vi "SoundCalibration.vi"(9 "通道号":i32, 10 "通道选择":enum16{"通道1", "通道2", "通道3", "通道4"}(ring), 11 "设备选择":refnum<visa-resource-name>) -> ()   [LabVIEW 2020, in "bas_meas.lvlib"]
uses:
  bas_meas.lvlib
panel:
  in  "取消":bool
  out "已排序的数组":string[](array[string])
  out "选中通道":string
  out "校准状态":string
  out "x-y":dbl
  out "数值":dbl
  out "结果字符串":string
  out "read buffer":string
  in  "校准声级(dB)":dbl=94.0 format="%.2g"
  out "SPL(dB)":dbl format="%.2f"
  in  "校准":bool
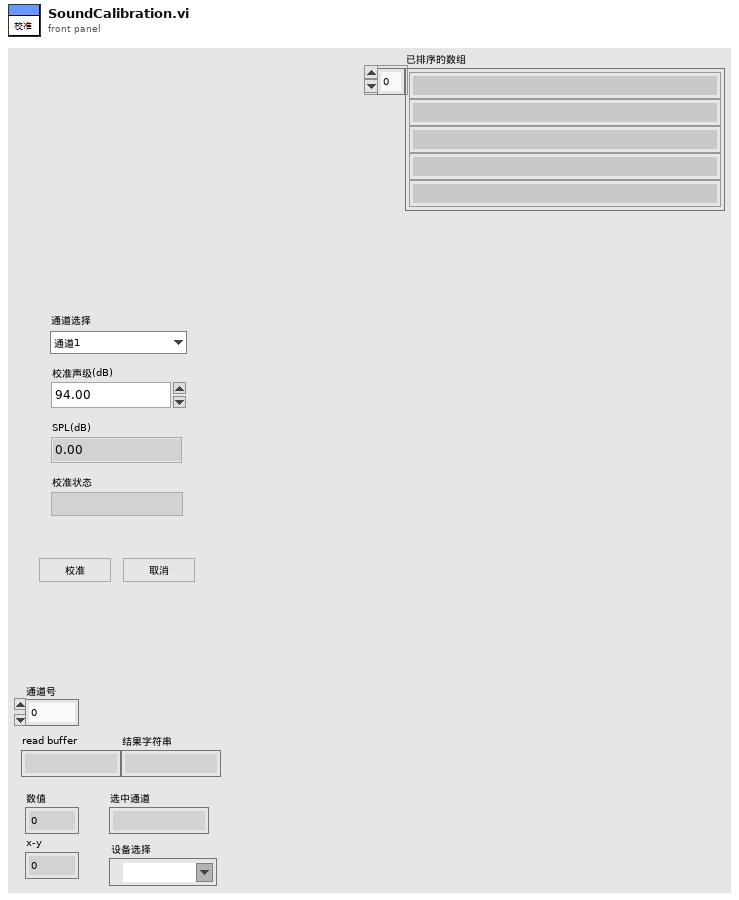
[diagram p1: front panel]
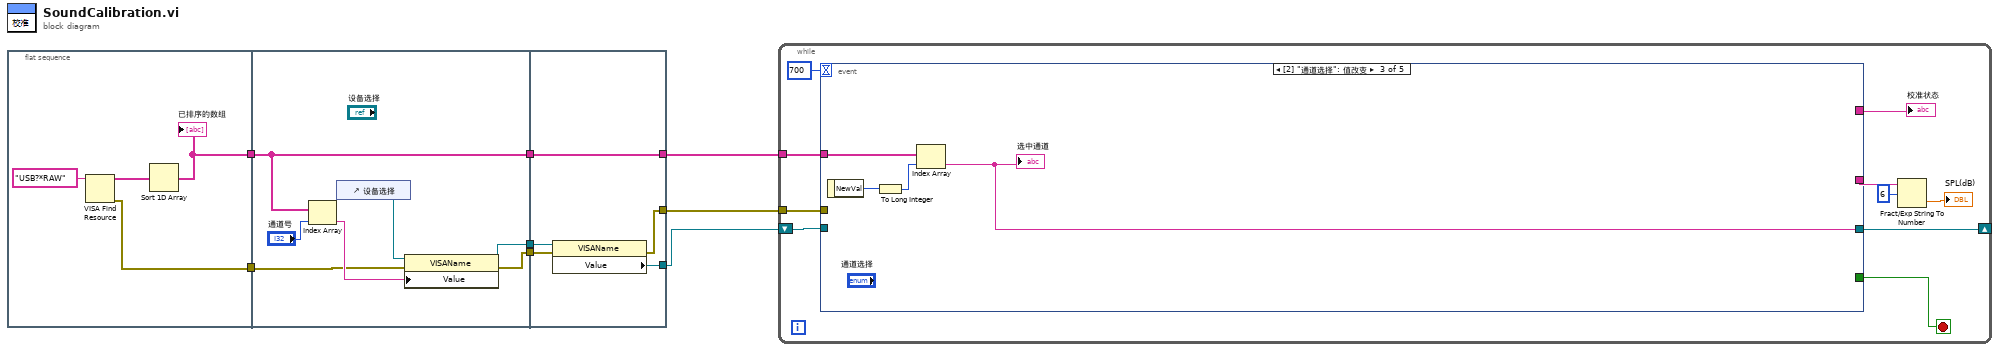
[diagram p0: block diagram]
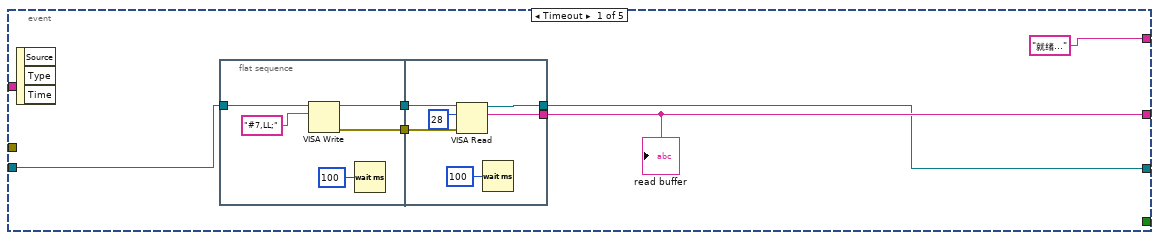
[diagram p2: hidden frame]
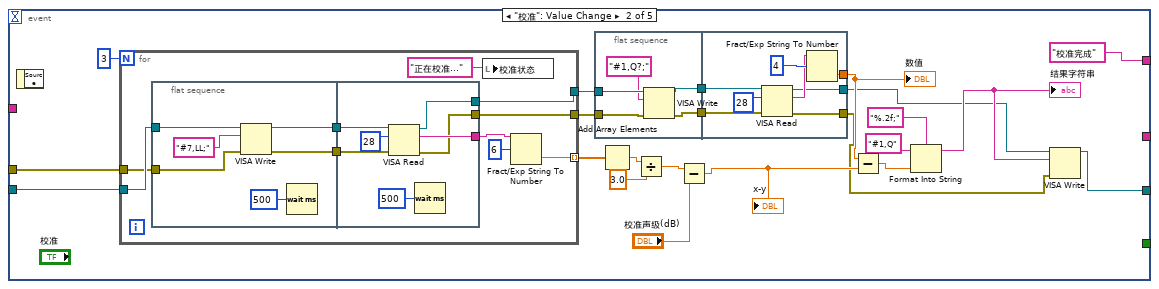
[diagram p3: hidden frame]
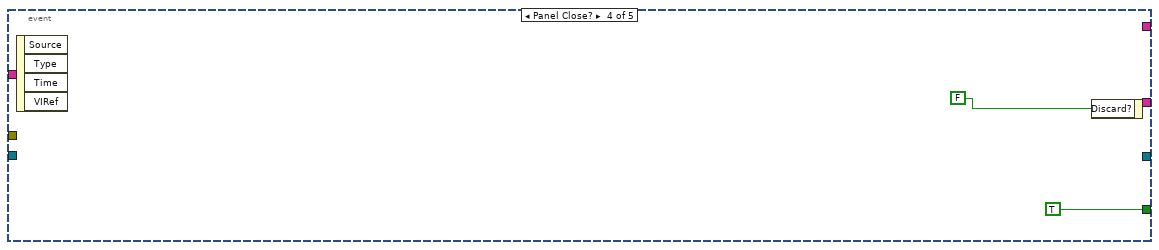
[diagram p4: hidden frame]
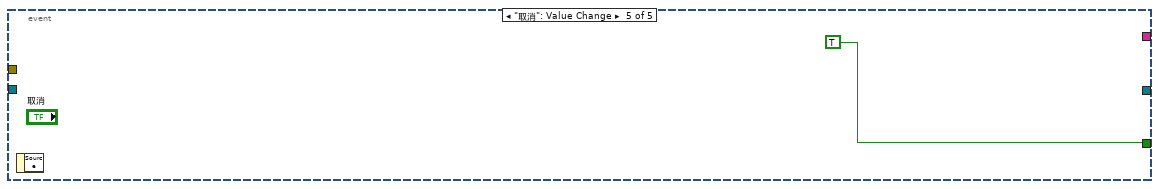
[diagram p5: hidden frame]
diagram:
  n1 = flat-sequence {
    tunnel: [w10] -> w7
    tunnel: [w9] -> w2
    tunnel: w7 -> [w19]
    tunnel: [w19] -> w6
    tunnel: [w16] -> w5
    tunnel: [w15] -> w4
    tunnel: w2 -> [w14]
    tunnel: [w24] -> w8
    tunnel: w6 -> [w24]
    tunnel: w5 -> [w23]
    tunnel: w4 -> [w22]
    tunnel: [w21] -> w3
    tunnel: [w20] -> w1
    frame #0 {
      n2 = VISA Find Resource(11:"USB?*RAW" ("表达式(\"?*\")")) -> (0:w9:errorcluster, 3:w11:string[])  [unwired: 2 in, 1 out]
      n3 = Sort 1D Array(array=w11) -> (sorted array=w10:string[])
      "已排序的数组" <- w10
    }
    frame #1 {
      n4 = Index Array(array=w19, index="通道号") -> (element=w18:string)
      n5 = control-ref of="设备选择"() -> (w17:refnum<vi>)
      n6 = property class="VISAName"(reference=w17, error in=w14, "Value"=w18) -> (reference out=w16:refnum<vi>, error out=w15:errorcluster)
    }
    frame #2 {
      n7 = property class="VISAName"(reference=w23, error in=w22) -> (error out=w20:errorcluster, "Value"=w21:refnum<visa-resource-name>)  [unwired: 1 out]
    }
  }
  n8 = while {
    tunnel: w8 -> [w27]
    shift-right: [w26] -> _
    shift-left: w3 -> [w33]
    tunnel: w1 -> [w25]
    stop <- w34 stop-if-true
    n9 = event shown="[2] \"通道选择\": 值改变" {
      selector: _ -> [_ _ _ _ _]
      dyn-events: _ -> [_ _ _ _ _]
      timeout: 700 -> [_ _ _ _ _]
      tunnel: [_ _ _ TRUE ("放弃？") TRUE ("放弃？")] -> w34
      tunnel: w33 -> [w38 w73 _ _ _]
      tunnel: [w37 _ _ _ _] -> w31
      tunnel: ["就绪..." "校准完成" _ _ _] -> w28
      tunnel: w27 -> [_ _ w113 _ _]
      tunnel: [w35 w53 w110 _ _] -> w26
      tunnel: w25 -> [_ w52 _ _ _]
      event Timeout {
        n10 = event-data() -> ()  [unwired: 1 in, 3 out]
        n11 = flat-sequence {
          tunnel: w38 -> [w45]
          tunnel: [w44] -> w40
          tunnel: [w43] -> w39
          tunnel: w40 -> [w51]
          tunnel: w39 -> [w50]
          tunnel: [w49] -> w37
          tunnel: [w46] -> w35
          frame #0 {
            n12 = VISA Write(VISA resource name=w45, write buffer="#7,LL;" ("写入缓冲区")) -> (VISA resource name out=w44:refnum<visa-resource-name>, error out=w43:errorcluster)  [unwired: 1 in, 1 out]
            n13 = Wait (ms)(milliseconds to wait=u32 100 ("等待时间（毫秒）")) -> ()  [unwired: 1 out]
          }
          frame #1 {
            n14 = VISA Read(VISA resource name=w51, byte count=u32 28 ("字节总数"), error in (no error)=w50) -> (VISA resource name out=w46:refnum<visa-resource-name>, read buffer=w49:string)  [unwired: 2 out]
            n15 = Wait (ms)(milliseconds to wait=u32 100 ("等待时间（毫秒）")) -> ()  [unwired: 1 out]
          }
        }
        "read buffer" <- w37
      }
      event "校准": Value Change {
        n16 = event-data() -> ()  [unwired: 1 in, 1 out]
        n17 = for {
          N: 3 -> [_]
          tunnel: w73 -> [w94]
          tunnel: [w91] -> w71 mode=indexing
          tunnel: [w90] -> w66
          tunnel: [w89] -> w65
          tunnel: w52 -> [w87]
          n18 = flat-sequence {
            tunnel: w94 -> [w102]
            tunnel: [w101] -> w96
            tunnel: [w100] -> w95
            tunnel: w87 -> [w97]
            tunnel: w96 -> [w109]
            tunnel: w95 -> [w108]
            tunnel: [w107] -> w92
            tunnel: [w104] -> w90
            tunnel: [w103] -> w89
            frame #0 {
              n19 = VISA Write(VISA resource name=w102, write buffer="#7,LL;" ("写入缓冲区"), error in (no error)=w97) -> (VISA resource name out=w101:refnum<visa-resource-name>, error out=w100:errorcluster)  [unwired: 1 out]
              n20 = Wait (ms)(milliseconds to wait=u32 500 ("等待时间（毫秒）")) -> ()  [unwired: 1 out]
            }
            frame #1 {
              n21 = VISA Read(VISA resource name=w109, byte count=u32 28 ("字节总数"), error in (no error)=w108) -> (VISA resource name out=w104:refnum<visa-resource-name>, read buffer=w107:string, error out=w103:errorcluster)  [unwired: 1 out]
              n22 = Wait (ms)(milliseconds to wait=u32 500 ("等待时间（毫秒）")) -> ()  [unwired: 1 out]
            }
          }
          n23 = local write "校准状态"("正在校准...") -> ()
          n24 = Fract/Exp String To Number(string=w92, offset=6 ("偏移量")) -> (number=w91:dbl)  [unwired: 2 in, 1 out]
        }
        n25 = flat-sequence {
          tunnel: w66 -> [w78]
          tunnel: w65 -> [w77]
          tunnel: [w75] -> w64
          tunnel: [w74] -> w63
          tunnel: w64 -> [w85]
          tunnel: w63 -> [w84]
          tunnel: [w81] -> w62
          tunnel: [w80] -> w56
          tunnel: [w79] -> w55
          frame #0 {
            n26 = VISA Write(VISA resource name=w78, write buffer="#1,Q?;" ("写入缓冲区"), error in (no error)=w77) -> (VISA resource name out=w75:refnum<visa-resource-name>, error out=w74:errorcluster)  [unwired: 1 out]
          }
          frame #1 {
            n27 = VISA Read(VISA resource name=w85, byte count=u32 28 ("字节总数"), error in (no error)=w84) -> (VISA resource name out=w80:refnum<visa-resource-name>, read buffer=w82:string, error out=w79:errorcluster)  [unwired: 1 out]
            n28 = Fract/Exp String To Number(string=w82, offset=4 ("偏移量")) -> (number=w81:dbl)  [unwired: 2 in, 1 out]
          }
        }
        n29 = Add Array Elements(numeric array=w71) -> (sum=w70:dbl)
        n30 = Divide(x=w70, y=3.0) -> (x/y=w68:dbl)
        n31 = Subtract(x=w68, y="校准声级(dB)") -> (x-y=w61:dbl)
        "x-y" <- w61
        n32 = Subtract(x=w62, y=w61) -> (x-y=w60:dbl)
        n33 = Format Into String(format string="%.2f;" ("格式字符串"), initial string="#1,Q" ("初始字符串"), w60) -> (resulting string=w57:string)  [unwired: 1 in, 1 out]
        "结果字符串" <- w57
        n34 = VISA Write(VISA resource name=w56, write buffer=w57, error in (no error)=w55) -> (VISA resource name out=w53:refnum<visa-resource-name>)  [unwired: 2 out]
        "数值" <- w62
      }
      event "通道选择": Value Change {
        n35 = event-data() -> ("NewVal"=w112:enum16{"通道1", "通道2", "通道3", "通道4"})  [unwired: 1 in]
        n36 = To Long Integer(number=w112) -> (32bit integer=w111:i32)
        n37 = Index Array(array=w113, index=w111) -> (element=w110:string)
        "选中通道" <- w110
      }
      event Panel Close? {
        n38 = event-data() -> ()  [unwired: 1 in, 4 out]
        n39 = event-data("Discard?"=FALSE ("放弃？")) -> ()  [unwired: 1 in, 1 out]
      }
      event "取消": Value Change {
        n40 = event-data() -> ()  [unwired: 1 in, 1 out]
      }
    }
    "校准状态" <- w28
    n41 = Fract/Exp String To Number(string=w31, offset=6 ("偏移量")) -> (number=→"SPL(dB)":dbl)  [unwired: 2 in, 1 out]
  }
